vi "Transmit.vi"(8 "error in (no error)":errorcluster, 9 "timeout in ms (-1)":i32=-1, 10 "Packet":refnum<class "Packet.lvclass">, 11 "Communication In":refnum<class "Local.lvclass">) -> (0 "error out":errorcluster, 1 "Timeout?":bool, 2 "Packet Sent":refnum<class "Packet.lvclass">, 3 "Communication Out":refnum<class "Local.lvclass">)   [LabVIEW 2020, in "Communication Classes.lvlib" / "Local.lvclass"]
uses:
  Local.lvclass
  IP_Communication/IP_Communication.lvclass
  Packet/Packet.lvclass
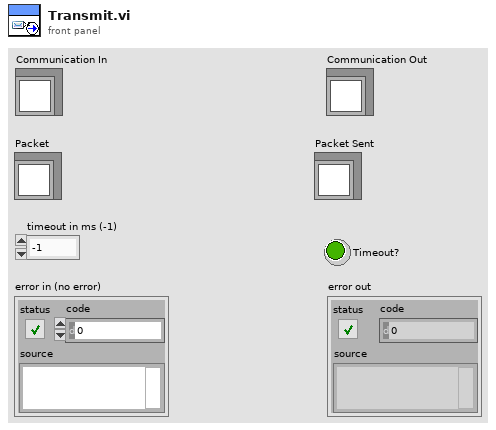
[diagram p1: front panel]
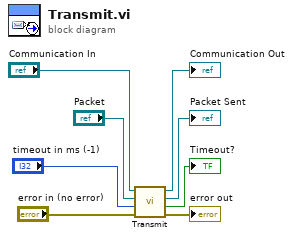
[diagram p0: block diagram]
diagram:
  n1 = call-parent "Transmit.vi"("error in (no error)"="error in (no error)", "timeout in ms (-1)"="timeout in ms (-1)", "Packet"="Packet", "Communication In"="Communication In") -> ("error out"=→"error out":errorcluster, "Timeout?"=→"Timeout?":bool, "Packet Sent"=→"Packet Sent":refnum<class "Packet.lvclass">, "Communication Out"=→"Communication Out":refnum<class "Local.lvclass">)  [unwired: 4 in]
